vi "4155C Shutdown.vi"(0 "VISA resource name in":refnum<visa-resource-name>, 3 "error in (no error)":errorcluster) -> (6 "error out":errorcluster)   [LabVIEW 2016]
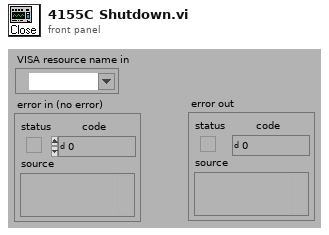
[diagram p1: front panel]
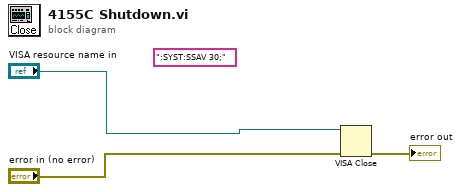
[diagram p0: block diagram]
diagram:
  (unwired) ":SYST:SSAV 30;" ("write buffer (\"\")")
  n1 = VISA Close(VISA resource name="VISA resource name in", error in (no error)="error in (no error)") -> (error out=→"error out":errorcluster)
